vi "Template Information Cache.vi"(8 "error in (no error)":errorcluster, 11 "Word_Report in":refnum<class "Word_Report.lvclass">) -> (0 "error out":errorcluster, 3 "Word_Report out":refnum<class "Word_Report.lvclass">)   [LabVIEW 2018, in "WordReportGeneration.lvlib" / "Word_Report.lvclass"]
uses:
  Word_Report.lvclass
  C:/Program Files (x86)/National Instruments/LabVIEW 2018/vi.lib/Utility/NIReport.llb/NI_report.lvclass
  Word_Report.lvclass/Word_Report.ctl
  WordReportGeneration.lvlib
  <vilib>/Utility/NIReport.llb/Word/NI_Word.lvclass
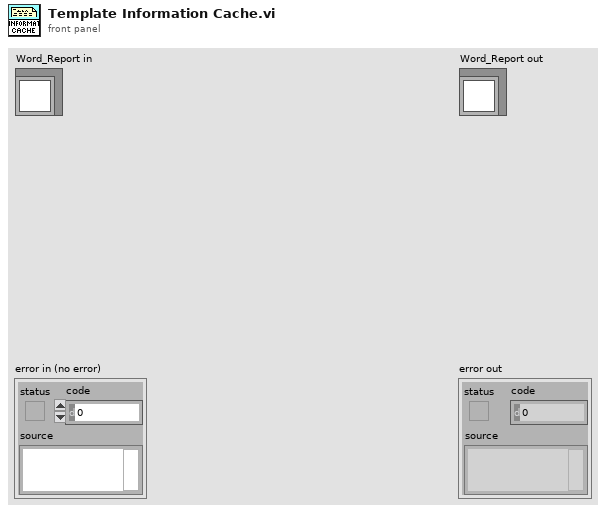
[diagram p1: front panel]
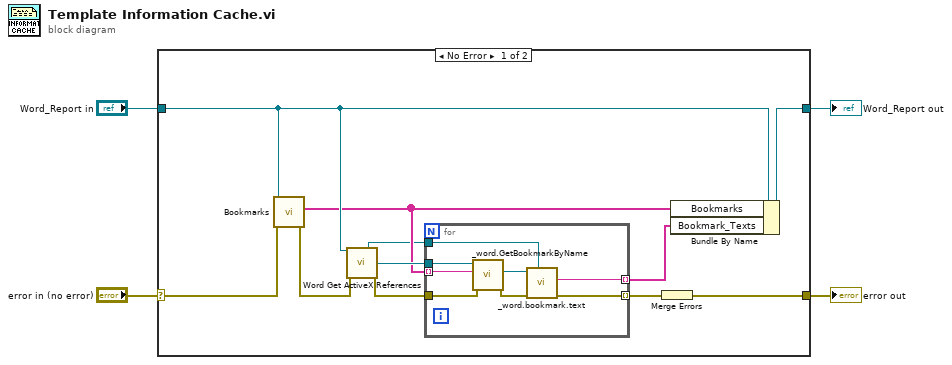
[diagram p0: block diagram]
diagram:
  n1 = case shown="No Error" "error in (no error)" {
    selector: "error in (no error)" -> [w14 w25]
    tunnel: [w5 w25] -> w3
    tunnel: [w15 w24] -> w1
    tunnel: "Word_Report in" -> [w13 w24]
    frame No Error {
      n2 = call "Bookmarks.vi"("error in (no error)"=w14, "NI_report in"=w13) -> ("error out"=w7:errorcluster, "Array"=w11:string[])  [unwired: 7 in, 1 out]
      n3 = call <vilib>:"Word Get ActiveX References.vi"("report in"=w13, "error in (no error)"=w7) -> ("Word._Application"=w10:refnum<k7>, "Word._Document"=w12:refnum<k7>, "error out"=w8:errorcluster)  [unwired: 7 in, 4 out]
      n4 = for {
        tunnel: w12 -> [w23]
        tunnel: w11 -> [w22] mode=indexing
        tunnel: w10 -> [w20]
        tunnel: [w19] -> w9 mode=indexing
        tunnel: w8 -> [w17]
        tunnel: [w16] -> w6 mode=indexing
        n5 = call "_word.GetBookmarkByName.vi"("error in (no error)"=w17, "String"=w22, "Document"=w23) -> ("error out"=w18:errorcluster, "bookmark"=w21:refnum<k7>)  [unwired: 5 in, 2 out]
        n6 = call "_word.bookmark.text.vi"("Application"=w20, "error IO"=w18, "Bookmark"=w21) -> ("error out"=w16:errorcluster, "Text"=w19:string)  [unwired: 6 in, 1 out]
      }
      n7 = Merge Errors(w6) -> (w5:errorcluster)
      n8 = Bundle By Name(cluster=w13, "Bookmarks"=w11, "Bookmark_Texts"=w9) -> (w15:refnum<class "Word_Report.lvclass">)
    }
    frame Error {
    }
  }
  "error out" <- w3
  "Word_Report out" <- w1
